vi "convert_step_vs_turn.vi"(8 "bypass_valve_turn_in":dbl, 9 "bypass_valve_step_in":i32, 10 "run_valve_turn_in":dbl, 11 "run_valve_step_in":i32) -> (0 "bypass_valve_step_out":i32, 1 "bypass_valve_turn_out":dbl, 2 "run_valve_step_out":i32, 3 "run_valve_turn_out":dbl)   [LabVIEW 2019]
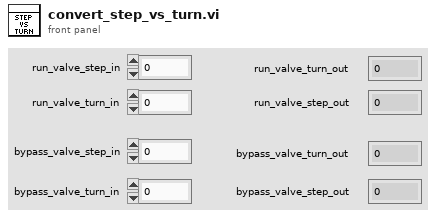
[diagram p1: front panel]
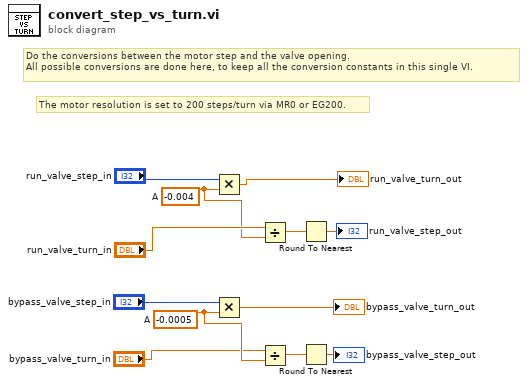
[diagram p0: block diagram]
diagram:
  w5 = -0.0005  # A
  w9 = -0.004  # A
  # "The motor resolution is set to 200 steps/turn via MR0 or EG200."
  # "Do the conversions between the motor step and the valve opening.\nAll possible conversions are done here, to keep all the conversion constants in this single VI."
  n1 = Multiply(x="run_valve_step_in", y=w9) -> (x*y=→"run_valve_turn_out":dbl)
  n2 = Multiply(x="bypass_valve_step_in", y=w5) -> (x*y=→"bypass_valve_turn_out":dbl)
  n3 = Divide(x="run_valve_turn_in", y=w9) -> (x/y=w7:dbl)
  n4 = Divide(x="bypass_valve_turn_in", y=w5) -> (x/y=w4:dbl)
  n5 = Round To Nearest(number=w7) -> (nearest integer value=→"run_valve_step_out":dbl)
  n6 = Round To Nearest(number=w4) -> (nearest integer value=→"bypass_valve_step_out":dbl)
